vi "Battery_Create.vi"(0 "reference in":refnum<class "Battery.lvclass">, 1 "Python venv":path=path "C:/Repo/volta-control-suite/venv", 2 "Python module":path=path "C:/Repo/volta-control-suite/src/Python/hps17k-pybamm-wrapper.py", 4 "Power Module":refnum<class "PowerModuleInterface.lvclass">, 5 "Error In":errorcluster, 6 "# Cells in Series":u16, 8 "# Cells in Parallel":u16) -> (14 "reference out":refnum<class "Battery.lvclass">, 15 "ProcessViRef":refnum<vi>, 19 "Error Out":errorcluster)   [LabVIEW 2023, in "Battery.lvclass"]
uses:
  Battery.lvclass
  builds/PowerModuleInterface/PowerModuleInterface.lvlibp/Classes/PowerModule_interface/PowerModuleInterface.lvclass
  <vilib>/Python/Open Venv Python Session.vi
  Battery.lvclass/Battery.ctl
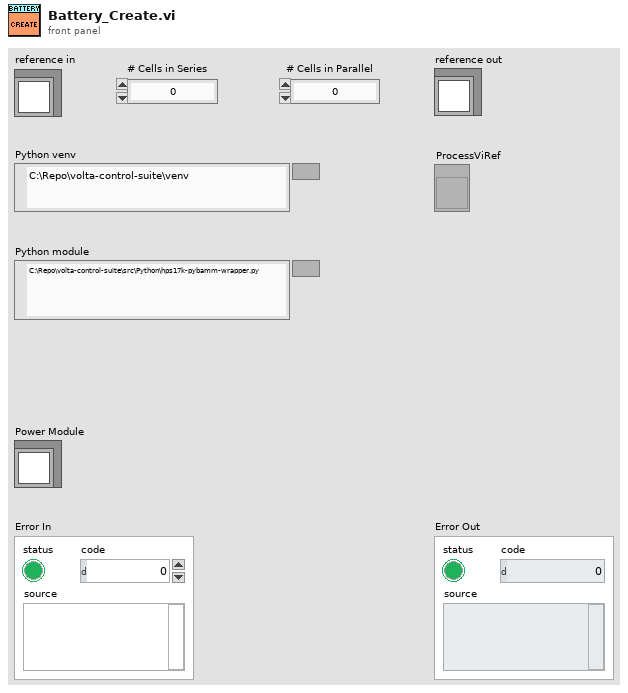
[diagram p1: front panel]
types:
  T1 = typedef "Battery.lvclass/ObjectAttributes.ctl" = cluster{"Python module":path, "Python Session":refnum<k35>, "PybammWrapper":refnum<k38>, "simulation loaded":bool, "simulation enabled":bool, "SOC OCV Curve":dbl[][], "Open Circuit Voltage (V)":dbl, "Terminal Voltage (V)":dbl, "State of Charge (%)":dbl, "# Cells in Series":u16, "# Cells in Parallel":u16, "Simulation Parameters":T2, "Power Module":refnum<class "PowerModuleInterface.lvclass">}
  T2 = typedef "Battery.lvclass/Simulation Parameters.ctl" = cluster{"num_rc_pairs":i32, "R0":dbl, "R1":dbl, "C1":dbl, "R2":dbl, "C2":dbl, " nominal_capacity_Ah":dbl, "upper_voltage_cutoff":dbl, "lower_voltage_cutoff":dbl}
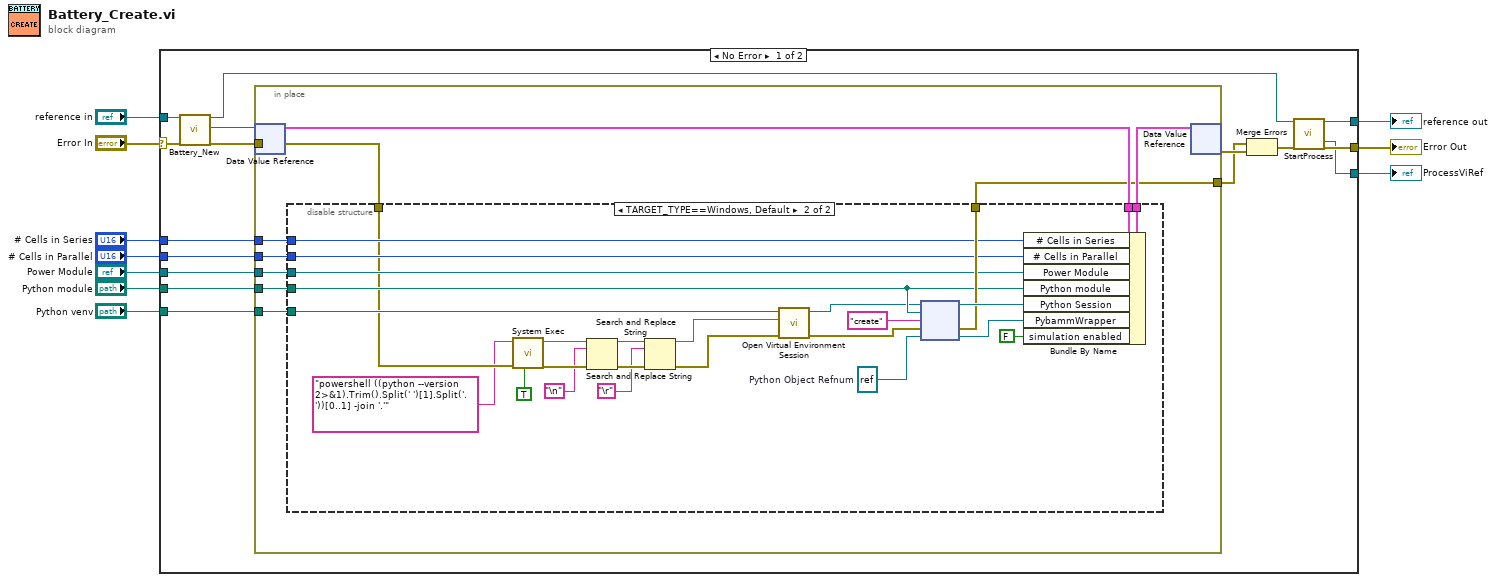
[diagram p0: block diagram]
diagram:
  n1 = case shown="No Error" "Error In" {
    selector: "Error In" -> [w25 w63]
    tunnel: [w18 w63] -> w9
    tunnel: "reference in" -> [w26 w62]
    tunnel: [w20 w62] -> w7
    tunnel: [w17 _] -> w6
    tunnel: "Python venv" -> [w11 _]
    tunnel: "Python module" -> [w16 _]
    tunnel: "Power Module" -> [w15 _]
    tunnel: "# Cells in Series" -> [w14 _]
    tunnel: "# Cells in Parallel" -> [w13 _]
    frame No Error {
      n2 = call "Battery_New.vi"("reference in"=w26, "Error In"=w25) -> ("reference out"=w21:refnum<class "Battery.lvclass">, "DVRRefOut"=w23:refnum<data-value>, "Error Out"=w12:errorcluster)  [unwired: 14 in, 1 out]
      n3 = in-place {
        in-place-border: [w33] -> w22
        in-place-border: w16 -> [w32]
        in-place-border: w15 -> [w29]
        in-place-border: w14 -> [w31]
        in-place-border: w13 -> [w30]
        in-place-border: w12 -> [w28]
        in-place-border: w11 -> [w27]
        n4 = in-place-dvr #1(w23) -> (w34:T1)  [unwired: 1 out]
        n5 = disable-structure shown="TARGET_TYPE==Windows, Default" {
          disable-tunnel: [_ w61] -> w35
          disable-tunnel: w34 -> [_ w60]
          disable-tunnel: [_ w55] -> w33
          disable-tunnel: w32 -> [_ w54]
          disable-tunnel: w31 -> [_ w53]
          disable-tunnel: w30 -> [_ w52]
          disable-tunnel: w29 -> [_ w51]
          disable-tunnel: w28 -> [_ w47]
          disable-tunnel: w27 -> [_ w50]
          frame condition #0 {
          }
          frame condition #1 (active) {
            w58 = refnum<k38> refnum  # Python Object Refnum
            n6 = call <vilib>:"System Exec.vi"("run minimized? (F)"=TRUE, "error in (no error)"=w47, "command line"="powershell ((python --version 2>&1).Trim().Split(' ')[1].Split('.'))[0..1] -join '.'") -> ("error out"=w39:errorcluster, "standard output"=w43:string)  [unwired: 5 in, 2 out]
            n7 = Search and Replace String(input string=w43, search string="\n", error in=w39) -> (result string=w44:string, error out=w40:errorcluster)  [unwired: 5 in, 2 out]
            n8 = Search and Replace String(input string=w44, search string="\r", error in=w40) -> (result string=w42:string, error out=w41:errorcluster)  [unwired: 5 in, 2 out]
            n9 = call-poly <vilib>:"Open Virtual Environment Session.vi"("error in (no error)"=w41, "Python version"=w42, "Env path"=w50) -> ("error out"=w49:errorcluster, "session out"=w48:refnum<k35>)  [unwired: 7 in]
            n10 = node(w48, w54, "create" ("function name"), w49, w58) -> (w57:refnum<k35>, w55:errorcluster, w56:refnum<k38>)  [unwired: 2 out]
            n11 = Bundle By Name(cluster=w60, "# Cells in Series"=w53, "# Cells in Parallel"=w52, "Power Module"=w51, "Python module"=w54, "Python Session"=w57, "PybammWrapper"=w56, "simulation enabled"=FALSE) -> (w61:T1)
          }
        }
        n12 = in-place-dvr #1(w35) -> (w24:errorcluster)  [unwired: 1 out]
      }
      n13 = Merge Errors(w22, w24) -> (w19:errorcluster)
      n14 = call "StartProcess.vi"("reference in"=w21, "Error In"=w19) -> ("reference out"=w20:refnum<class "Battery.lvclass">, "ProcessViRef"=w17:refnum<vi>, "Error Out"=w18:errorcluster)  [unwired: 13 in, 2 out]
    }
    frame Error {
      # "VI-TechBaseTemplate_Simple_6x8x6"
    }
  }
  "Error Out" <- w9
  "reference out" <- w7
  "ProcessViRef" <- w6
